vi "SP_Exchange.vi"(8 "error in (no error)":errorcluster, 10 "command":string, 11 "SemiProbe in":refnum<class "SemiProbe.lvclass">) -> (0 "error out":errorcluster, 2 "answer":string, 3 "SemiProbe out":refnum<class "SemiProbe.lvclass">, 4 "return count read":u32, 5 "return count write":u32)   [LabVIEW 2019, in "SemiProbe.lvclass"]
uses:
  SemiProbe.lvclass
panel:
  out "Loops with same bytes at port":u32
  out "SP BUSY":bool
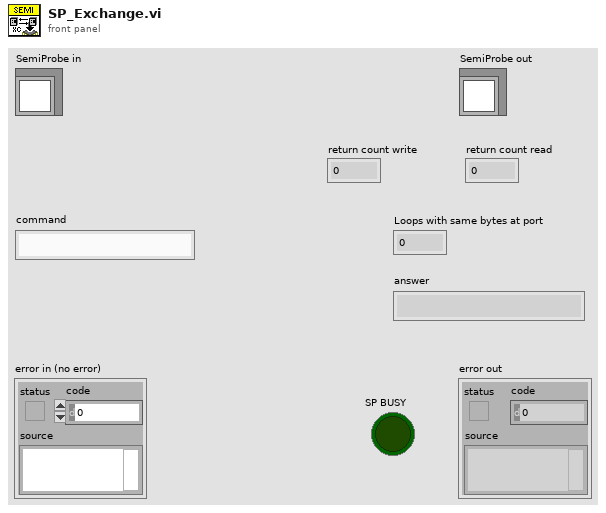
[diagram p1: front panel]
types:
  T1 = cluster{"SemiProbe VISA":refnum<visa-resource-name>, "write delay(ms)":i32, "buffer is full loop multiplicity":i32, "read threshold check rate (ms)":u32}
  T2 = cluster{"LF as Return EOL":bool, "SP Error Debug":bool}
  T3 = cluster{"address":string, "port":i32, "SP TCP Cnx ID":refnum<k5>, "mode (standard)":enum16{"Standard", "Buffered", "CRLF", "Immediate"}, "bytes to read":i32, "timeout (ms)":i32}
  T4 = enum16{"Standard", "Buffered", "CRLF", "Immediate"}
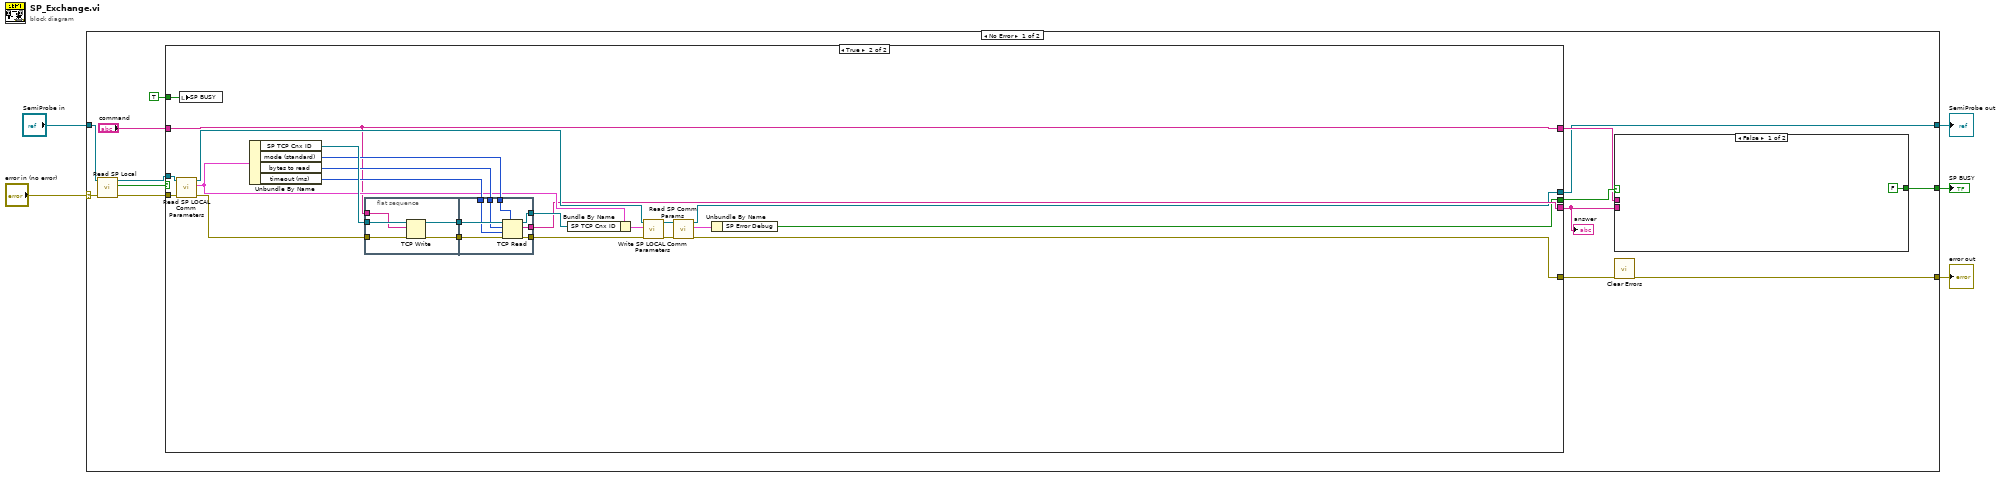
[diagram p0: block diagram]
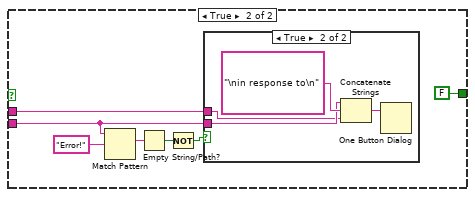
[diagram p2: hidden frame]
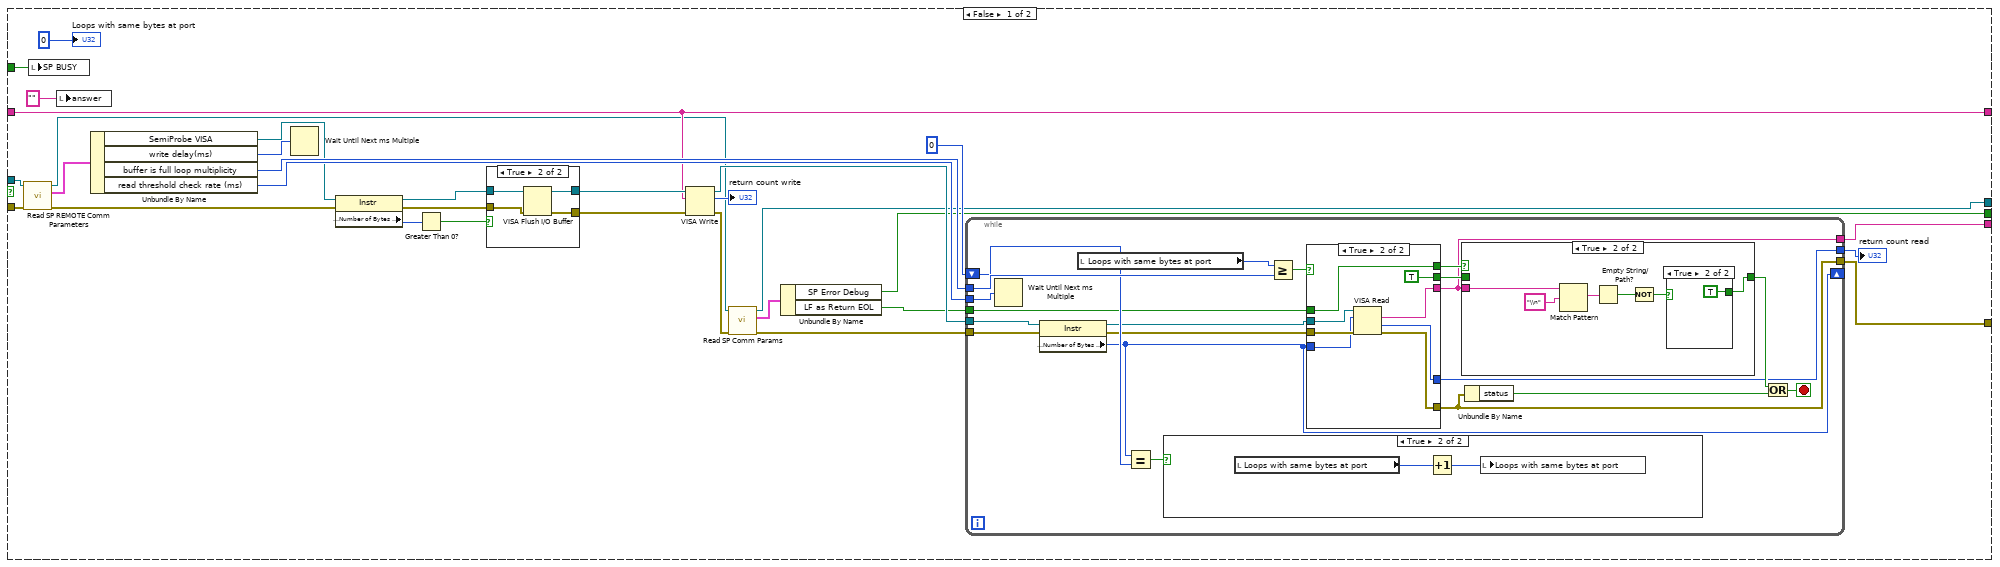
[diagram p4: hidden frame]
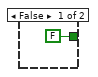
[diagram p6: hidden frame]
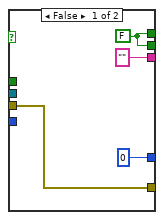
[diagram p7: hidden frame]
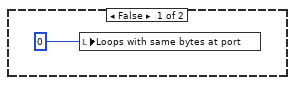
[diagram p8: hidden frame]
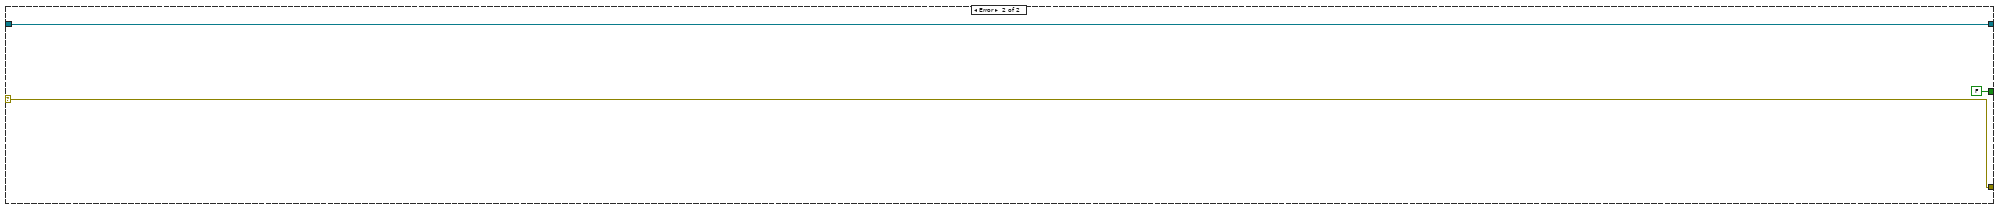
[diagram p10: hidden frame]
diagram:
  n1 = case shown="No Error" "error in (no error)" {
    selector: "error in (no error)" -> [w14 w151]
    tunnel: [w12 w151] -> w4
    tunnel: [w8 w150] -> w2
    tunnel: "SemiProbe in" -> [w19 w150]
    tunnel: [w6 FALSE] -> w1
    frame No Error {
      n2 = call-dynamic "Read SP Local.vi"("error in (no error)"=w14, "SemiProbe in"=w19) -> ("error out"=w15:errorcluster, "SP Local"=w18:bool, "SemiProbe out"=w16:refnum<class "SemiProbe.lvclass">)  [unwired: 7 in]
      n3 = case shown="True" w18 {
        tunnel: TRUE -> [w62 w135]
        tunnel: w16 -> [w34 w134]
        tunnel: w15 -> [w35 w133]
        tunnel: "command" -> [w41 w116]
        tunnel: [w43 w114] -> w11
        tunnel: [w40 w115] -> w10
        tunnel: [w42 w117] -> w7
        tunnel: [w41 w116] -> w9
        tunnel: [w39 w113] -> w8
        frame False {
          n4 = call-dynamic "Read SP REMOTE Comm Parameters.vi"("error in (no error)"=w35, "SemiProbe in"=w34) -> ("error out"=w37:errorcluster, "SP REMOTE Comm Parameters"=w54:T1, "SemiProbe out"=w33:refnum<class "SemiProbe.lvclass">)  [unwired: 7 in]
          n5 = local write "SP BUSY"(w62) -> ()
          n6 = local write "answer"("" ("answer")) -> ()
          n7 = Unbundle By Name(w54) -> ("SemiProbe VISA"=w36:refnum<visa-resource-name>, "write delay(ms)"=w53:i32, "buffer is full loop multiplicity"=w45:i32, "read threshold check rate (ms)"=w50:u32)
          n8 = Wait Until Next ms Multiple(millisecond multiple=w53) -> ()  [unwired: 1 out]
          n9 = property class="Instr"(reference=w36, error in=w37) -> (reference out=w58:refnum<visa-resource-name>, error out=w59:errorcluster, "Serial Settings:Number of Bytes at Serial Port"=w61:u32)
          n10 = Greater Than 0?(x=w61) -> (x > 0?=w60:bool)
          n11 = case shown="True" w60 {
            tunnel: w59 -> [w108 w112]
            tunnel: w58 -> [w107 w111]
            tunnel: [w108 w110] -> w57
            tunnel: [w107 w109] -> w56
            frame False {
            }
            frame True {
              n12 = VISA Flush I/O Buffer(VISA resource name=w111, error in (no error)=w112) -> (VISA resource name out=w109:refnum<visa-resource-name>, error out=w110:errorcluster)  [unwired: 1 in]
            }
          }
          n13 = VISA Write(VISA resource name=w56, write buffer=w41, error in (no error)=w57) -> (VISA resource name out=w47:refnum<visa-resource-name>, return count=→"return count write":u32, error out=w32:errorcluster)
          n14 = call-dynamic "Read SP Comm Params.vi"("error in (no error)"=w32, "SemiProbe in"=w33) -> ("error out"=w48:errorcluster, "SP Comm Params"=w49:T2, "SemiProbe out"=w39:refnum<class "SemiProbe.lvclass">)  [unwired: 7 in]
          n15 = Unbundle By Name(w49) -> ("SP Error Debug"=w40:bool, "LF as Return EOL"=w44:bool)
          n16 = while {
            tunnel: w50 -> [w82]
            tunnel: w48 -> [w81]
            tunnel: w47 -> [w80]
            shift-right: [w72] -> _
            shift-left: u32 0 -> [w77]
            tunnel: w45 -> [w78]
            tunnel: w44 -> [w71]
            tunnel: [w65] -> w43
            tunnel: [w64] -> w42
            tunnel: [w63] -> w38
            stop <- w69 stop-if-true
            n17 = Wait Until Next ms Multiple(millisecond multiple=w82) -> ()  [unwired: 1 out]
            n18 = property class="Instr"(reference=w80, error in=w81) -> (reference out=w73:refnum<visa-resource-name>, error out=w74:errorcluster, "Serial Settings:Number of Bytes at Serial Port"=w72:u32)
            n19 = local read "Loops with same bytes at port"() -> (w79:u32)
            n20 = Equal?(x=w72, y=w77) -> (x = y?=w76:bool)
            n21 = case shown="True" w76 {
              frame False {
                n22 = local write "Loops with same bytes at port"(0) -> ()
              }
              frame True {
                n23 = local read "Loops with same bytes at port"() -> (w106:u32)
                n24 = Increment(x=w106) -> (x+1=w105:u32)
                n25 = local write "Loops with same bytes at port"(w105) -> ()
              }
            }
            n26 = Greater Or Equal?(x=w79, y=w78) -> (x >= y?=w75:bool)
            n27 = case shown="True" w75 {
              tunnel: w74 -> [w95 w103]
              tunnel: w73 -> [_ w102]
              tunnel: w72 -> [_ w101]
              tunnel: w71 -> [_ w100]
              tunnel: [w95 w96] -> w65
              tunnel: [u32 0 ("return count") w97] -> w63
              tunnel: [w92 w100] -> w68
              tunnel: ["" ("read buffer") w98] -> w64
              tunnel: [w92 TRUE] -> w67
              frame False {
                w92 = FALSE
              }
              frame True {
                n28 = VISA Read(VISA resource name=w102, byte count=w101, error in (no error)=w103) -> (read buffer=w98:string, return count=w97:u32, error out=w96:errorcluster)  [unwired: 1 out]
              }
            }
            n29 = case shown="True" w68 {
              tunnel: w64 -> [_ w86]
              tunnel: [w83 w84] -> w66
              tunnel: w67 -> [w83 _]
              frame False {
              }
              frame True {
                n30 = Match Pattern(string=w86, regular expression="\\n") -> (match substring=w89:string)  [unwired: 1 in, 3 out]
                n31 = Empty String/Path?(string/path=w89) -> (empty?=w88:bool)
                n32 = Not(x=w88) -> (.not. x?=w85:bool)
                n33 = case shown="True" w85 {
                  tunnel: [FALSE TRUE] -> w84
                  frame False {
                  }
                  frame True {
                  }
                }
              }
            }
            n34 = Unbundle By Name(w65) -> ("status"=w70:bool)
            n35 = Or(x=w66, y=w70) -> (x .or. y?=w69:bool)
          }
          "return count read" <- w38
          "Loops with same bytes at port" <- 0
        }
        frame True {
          n36 = call-dynamic "Read SP LOCAL Comm Parameters.vi"("error in (no error)"=w133, "SemiProbe in"=w134) -> ("error out"=w130:errorcluster, "SP LOCAL Comm Parameters"=w124:T3, "SemiProbe out"=w119:refnum<class "SemiProbe.lvclass">)  [unwired: 7 in]
          n37 = local write "SP BUSY"(w135) -> ()
          n38 = Unbundle By Name(w124) -> ("SP TCP Cnx ID"=w129:refnum<k5>, "mode (standard)"=w128:T4, "bytes to read"=w127:i32, "timeout (ms)"=w126:i32)
          n39 = flat-sequence {
            tunnel: w129 -> [w138]
            tunnel: w130 -> [w137]
            tunnel: [w140] -> w132
            tunnel: [w139] -> w131
            tunnel: w116 -> [w136]
            tunnel: [w146] -> w120
            tunnel: [w147] -> w125
            tunnel: w132 -> [w148]
            tunnel: w131 -> [w145]
            tunnel: w128 -> [w144]
            tunnel: w127 -> [w143]
            tunnel: w126 -> [w142]
            tunnel: [w141] -> w117
            frame #0 {
              n40 = TCP Write(connection ID=w138, data in=w136, error in (no error)=w137) -> (connection ID out=w140:refnum<k5>, error out=w139:errorcluster)  [unwired: 2 out]
            }
            frame #1 {
              n41 = TCP Read(connection ID=w148, bytes to read=w143, error in (no error)=w145, 7:w144, 9:w142) -> (connection ID out=w147:refnum<k5>, data out=w141:string, error out=w146:errorcluster)
            }
          }
          n42 = Bundle By Name(cluster=w124, "SP TCP Cnx ID"=w125) -> (w122:T3)
          n43 = call-dynamic "Write SP LOCAL Comm Parameters.vi"("error in (no error)"=w120, "SP LOCAL Comm Parameters"=w122, "SemiProbe in"=w119) -> ("error out"=w118:errorcluster, "SemiProbe out"=w121:refnum<class "SemiProbe.lvclass">)  [unwired: 7 in]
          n44 = call-dynamic "Read SP Comm Params.vi"("error in (no error)"=w118, "SemiProbe in"=w121) -> ("error out"=w114:errorcluster, "SP Comm Params"=w123:T2, "SemiProbe out"=w113:refnum<class "SemiProbe.lvclass">)  [unwired: 7 in]
          n45 = Unbundle By Name(w123) -> ("SP Error Debug"=w115:bool)
        }
      }
      "answer" <- w7
      n46 = case shown="False" w10 {
        tunnel: w7 -> [_ w21]
        tunnel: w9 -> [_ w23]
        tunnel: [FALSE FALSE] -> w6
        frame False {
        }
        frame True {
          n47 = Match Pattern(string=w21, regular expression="Error!") -> (match substring=w25:string)  [unwired: 1 in, 3 out]
          n48 = Empty String/Path?(string/path=w25) -> (empty?=w26:bool)
          n49 = Not(x=w26) -> (.not. x?=w24:bool)
          n50 = case shown="True" w24 {
            tunnel: w21 -> [_ w29]
            tunnel: w23 -> [_ w28]
            frame False {
            }
            frame True {
              n51 = Concatenate Strings(w29, "\nin response to\n" ("regular expression"), w28) -> (w31:string)
              n52 = One Button Dialog(message=w31) -> ()  [unwired: 1 in, 1 out]
            }
          }
        }
      }
      n53 = call <vilib>:"Clear Errors.vi"("error in (no error)"=w11) -> ("error out"=w12:errorcluster)  [unwired: 5 in, 1 out]
    }
    frame Error {
    }
  }
  "error out" <- w4
  "SemiProbe out" <- w2
  "SP BUSY" <- w1
